vi "RxDatos.vi"() -> ()   [LabVIEW 2020]
uses:
  <vilib>/httpClient/LabVIEWHTTPClient.lvlib
panel:
  out "Rele":bool
  out "Feedback[mA]":dbl
  out "Hora 2":string
  out "Hora":string
  out "Data":string
  out "error GET":errorcluster
  in  "stop":bool
  out "body GET":string
  out "headers GET":string
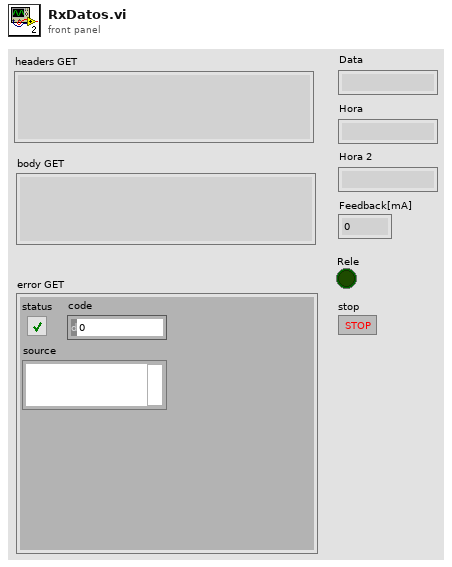
[diagram p1: front panel]
types:
  T1 = cluster{"Data":string, "Accionamiento":dbl, "Rele":bool, "Hora":string}
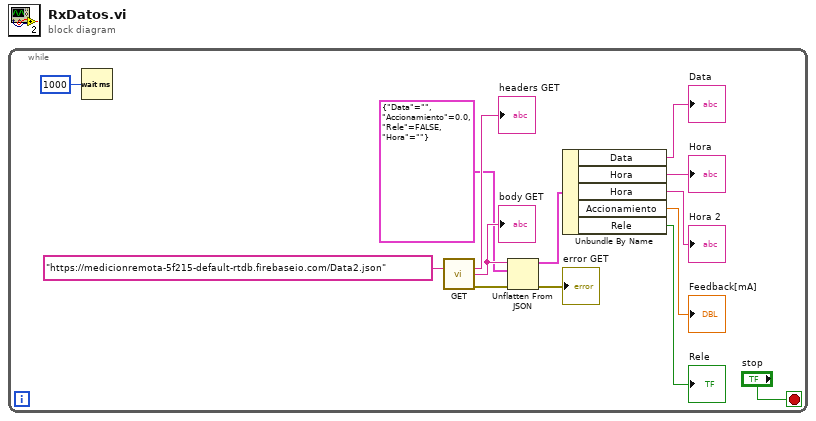
[diagram p0: block diagram]
diagram:
  n1 = while {
    stop <- "stop" stop-if-true
    n2 = Wait (ms)(milliseconds to wait=u32 1000) -> ()  [unwired: 1 out]
    n3 = call <vilib>:"GET.vi"("url"="https://medicionremota-5f215-default-rtdb.firebaseio.com/Data2.json") -> ("headers"=→"headers GET":string, "body"=w10:string, "error out"=w9:errorcluster)  [unwired: 11 in, 1 out]
    "body GET" <- w10
    n4 = Unflatten From JSON(JSON string=w10, type and defaults=T1 {"Data"="", "Accionamiento"=0.0, "Rele"=FALSE, "Hora"=""}, error in (no error)=w9) -> (value=w6:T1, error out=→"error GET":errorcluster)  [unwired: 4 in]
    n5 = Unbundle By Name(w6) -> ("Data"=→"Data":string, "Hora"=→"Hora":string, "Hora"=→"Hora 2":string, "Accionamiento"=→"Feedback[mA]":dbl, "Rele"=→"Rele":bool)
  }
